vi "Out_S7F1.vi"(8 "error in (no error)":errorcluster, 10 "S7F1":T1, 11 "S7 Message Class in":refnum<class "S7 Message Class.lvclass">) -> (0 "error out":errorcluster, 3 "S7 Message Class out":refnum<class "S7 Message Class.lvclass">)   [LabVIEW 2020, in "SECS Communication.lvlib" / "S7 Message Class.lvclass"]
uses:
  S7 Message Class.lvclass
  D:/Dropbox/SECS/LabVIEW Code/Com/SECS Communication/SECS-II Class/SECS-II Class.lvclass
  S7F1.ctl
  SECS-II Class/Data Message_List.vi
  SECS-II Class/Data Message_ASCII.vi
  SECS-II Class/Data Message_U4.vi
  S7 Message Class.lvclass/S7 Message Class.ctl
  SECS-II Class/SECS-II Class.lvclass
  D:/Dropbox/SECS/LabVIEW Code/Com/SECS Communication/S7 Message Class/S7 Message Class.lvclass
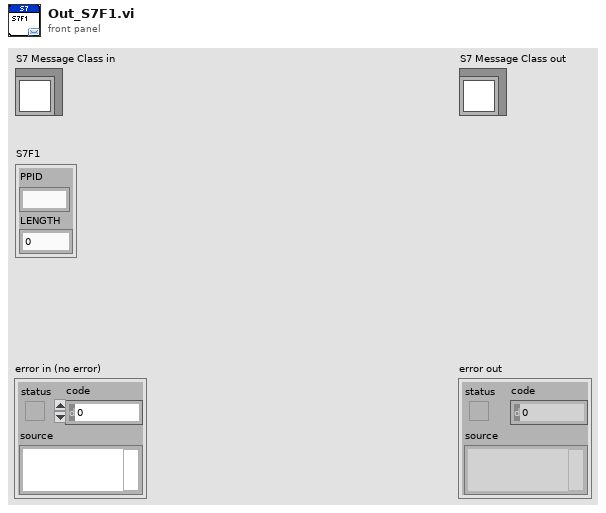
[diagram p1: front panel]
types:
  T1 = typedef "SECS Communication.lvlib/S7 Message Class.lvclass/S7F1.ctl" = cluster{"PPID":string, "LENGTH":u32}
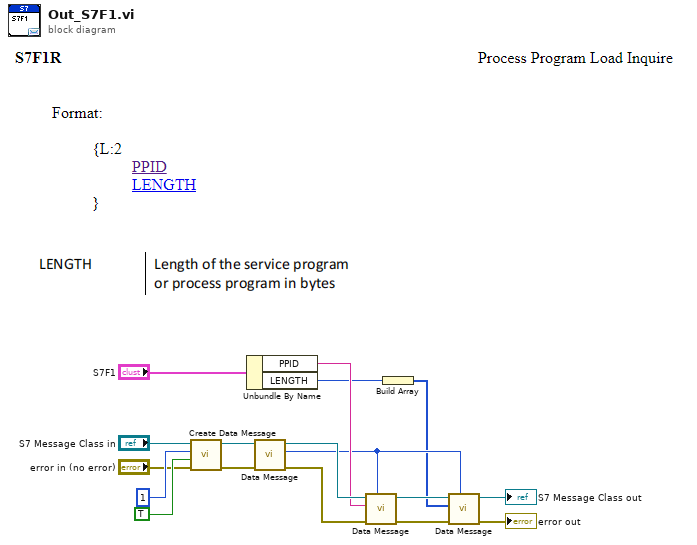
[diagram p0: block diagram]
diagram:
  n1 = call "Create Data Message.vi"("error in (no error)"="error in (no error)", "W-Bit"=TRUE, "Function"=u8 1, "SECS-II Class in"="S7 Message Class in") -> ("error out"=w6:errorcluster, "SECS-II Class out"=w7:refnum<class "S7 Message Class.lvclass">)  [unwired: 6 in]
  n2 = Unbundle By Name("S7F1") -> ("PPID"=w11:string, "LENGTH"=w2:u32)
  n3 = call-poly "Data Message.vi"("error in"=w6, "SECS-II Class in"=w7) -> ("error out"=w12:errorcluster, "Index"=w8:i32, "SECS-II Class out"=w13:refnum<class "S7 Message Class.lvclass">)  [unwired: 7 in]
  n4 = call-poly "Data Message.vi"("Parent Index"=w8, "error in"=w12, "Data"=w11, "SECS-II Class in"=w13) -> ("error out"=w9:errorcluster, "SECS-II Class out"=w10:refnum<class "S7 Message Class.lvclass">)  [unwired: 6 in]
  n5 = Build Array(w2) -> (w1:u32[])
  n6 = call-poly "Data Message.vi"("Parent Index"=w8, "error in"=w9, "Data"=w1, "SECS-II Class in"=w10) -> ("error out"=→"error out":errorcluster, "SECS-II Class out"=→"S7 Message Class out":refnum<class "S7 Message Class.lvclass">)  [unwired: 6 in]
